vi "LV Exp5.vi"() -> ()   [LabVIEW 2009]
uses:
  <vilib>/NXT/Block Support/NXT_InputPort.ctl
  <vilib>/NXT/Dual Mode Library/Display/drawText.vi
  <vilib>/NXT/Dual Mode Library/Waits/Wait_Num(msec).vi
panel:
  in  "stop":bool
  # "HiTechnic Experimenter's Kit\n\n                        Experiment 5 - Ambient Canceling Light sensor.\nThis program reads the photo cell on A0 with the LED off\nand again with the LED on, subtracts the level without the \nLED to cancel the background light level.\n\nSee Experimenter's Kit Handbook for the SuperPro for\nmore information or go to www.hitechnic.com.\n\n(c) HiTechnic 2011"
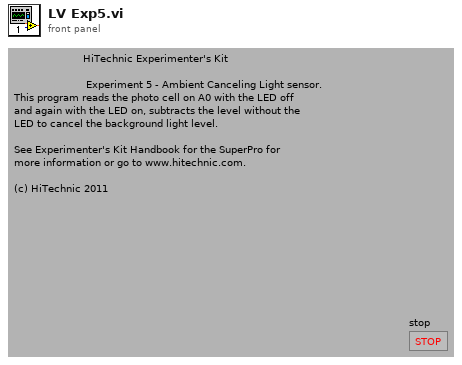
[diagram p1: front panel]
types:
  T1 = typedef "NXT_InputPort.ctl" = u8
  T2 = typedef "LVHSConnector.ctl" = cluster{"error":errorcluster, "address":string, "NXT #":i32, "Show Error":bool, "Connection":u16}
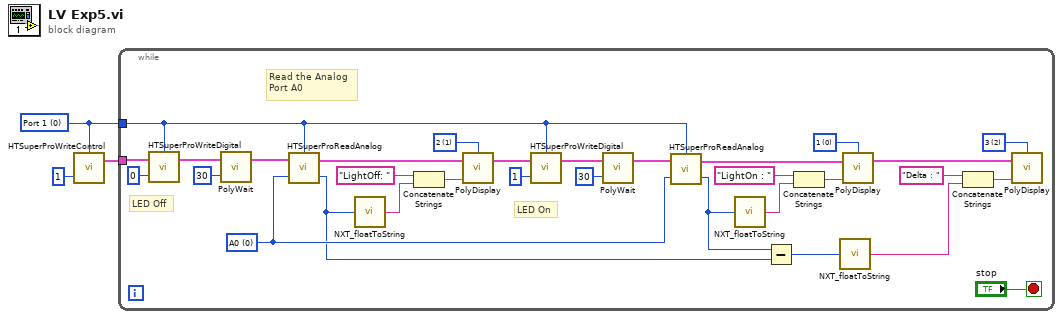
[diagram p0: block diagram]
diagram:
  w1 = T1 0 items=["Port 1", "Port 2", "Port 3", "Port 4"] ("Port")
  n1 = call "HTSuperProWriteControl.vi"("Digital Value"=u8 1, "Port"=w1) -> ("NXT"=w2:T2)  [unwired: 3 in]
  n2 = while {
    tunnel: w1 -> [w17]
    tunnel: w2 -> [w29]
    stop <- "stop" stop-if-true
    w9 = i16 2 items=["1", "2", "3", "4", "5", "6", "7", "8"] ("Line")
    w12 = i16 0 items=["1", "2", "3", "4", "5", "6", "7", "8"] ("Line")
    w24 = i16 1 items=["1", "2", "3", "4", "5", "6", "7", "8"] ("Line")
    w18 = u8 0 items=["A0", "A1", "A2", "A3"] ("Analog Port")
    # "LED On"
    # "LED Off"
    # "Read the Analog\nPort A0"
    n3 = call "HTSuperProWriteDigital.vi"("Digital Value"=u8 0, "NXT"=w29, "Port"=w17) -> ("NXT"=w27:T2)  [unwired: 2 in]
    n4 = call-poly <vilib>:"PolyWait.vi"("Time (100 msec)"=u32 30, "NXT"=w27) -> ("NXT"=w25:T2)  [unwired: 2 in]
    n5 = call "HTSuperProReadAnalog.vi"("Analog Port"=w18, "NXT"=w25, "Port"=w17) -> ("Analog Value"=w10:i16, "NXT"=w33:T2)  [unwired: 1 in]
    n6 = call <vilib>:"NXT_floatToString.vi"("number"=w10) -> ("string"=w30:string)
    n7 = Concatenate Strings("LightOff: " ("string"), w30) -> (w32:string)
    n8 = call-poly <vilib>:"PolyDisplay.vi"("Text"=w32, "NXT"=w33, "Line"=w24) -> ("NXT"=w19:T2)  [unwired: 1 in]
    n9 = call "HTSuperProWriteDigital.vi"("Digital Value"=u8 1, "NXT"=w19, "Port"=w17) -> ("NXT"=w21:T2)  [unwired: 2 in]
    n10 = call-poly <vilib>:"PolyWait.vi"("Time (100 msec)"=u32 30, "NXT"=w21) -> ("NXT"=w23:T2)  [unwired: 2 in]
    n11 = call "HTSuperProReadAnalog.vi"("Analog Port"=w18, "NXT"=w23, "Port"=w17) -> ("Analog Value"=w11:i16, "NXT"=w13:T2)  [unwired: 1 in]
    n12 = call <vilib>:"NXT_floatToString.vi"("number"=w11) -> ("string"=w16:string)
    n13 = Subtract(x=w11, y=w10) -> (x-y=w4:i16)
    n14 = Concatenate Strings("LightOn : " ("string"), w16) -> (w14:string)
    n15 = call <vilib>:"NXT_floatToString.vi"("number"=w4) -> ("string"=w6:string)
    n16 = call-poly <vilib>:"PolyDisplay.vi"("Text"=w14, "NXT"=w13, "Line"=w12) -> ("NXT"=w5:T2)  [unwired: 1 in]
    n17 = Concatenate Strings("Delta : " ("string"), w6) -> (w8:string)
    n18 = call-poly <vilib>:"PolyDisplay.vi"("Text"=w8, "NXT"=w5, "Line"=w9) -> ()  [unwired: 1 in, 1 out]
  }
